vi "stepper driver -- progress monitor.vi"(8 "talkback user event":refnum<user-event>, 11 "talkto user event":refnum<user-event>) -> ()   [LabVIEW 2018]
uses:
  stepper motor state.ctl
  stepper progress monitor message.ctl
  talkto async routine action.ctl
  stepper driver action.ctl
  stepper driver -- BLM.vi
  stepper driver -- IMS.vi
panel:
  in  "stepper state":T1=enum."stopped"
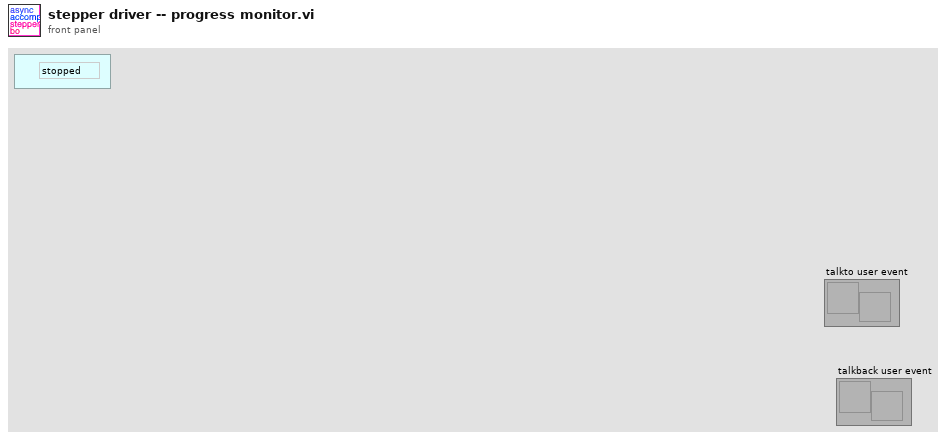
[diagram p1: front panel]
types:
  T1 = typedef "stepper motor state.ctl" = enum16{"moving", "stopped"}
  T2 = typedef "talkto async routine action.ctl" = enum16{"stop", "check"}
  T3 = typedef "stepper driver action.ctl" = enum16{"go", "void", "stop", "check", "init", "sync", "set", "set speed", "--check status", "--check value"}
  T4 = typedef "stepper progress monitor message.ctl" = cluster{"current position":dbl, "stepper motor state OUT":T1}
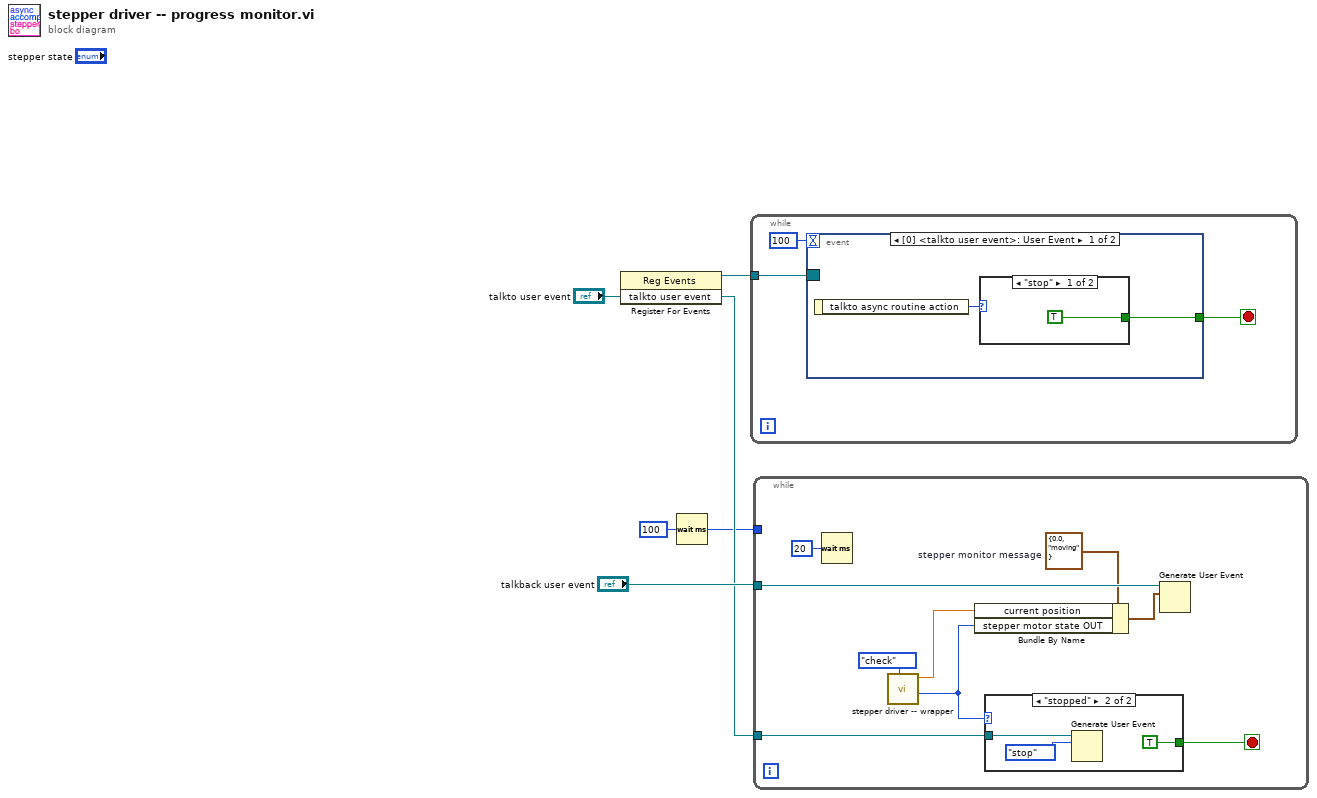
[diagram p0: block diagram]
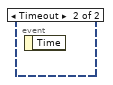
[diagram p3: hidden frame]
diagram:
  n1 = register-events("talkto user event") -> (reference out=w3:refnum<event-registration>)  [unwired: 2 in, 1 out]
  n2 = Wait (ms)(milliseconds to wait=u32 100) -> (millisecond timer value=w1:u32)
  n3 = while {
    tunnel: w3 -> [w8]
    stop <- w6 stop-if-true
    n4 = event shown="[0] <talkto user event>: User Event" {
      selector: w8 -> [_ _]
      dyn-events: _ -> [_ _]
      timeout: 100 -> [_ _]
      tunnel: [w9 _] -> w6
      event User Event {
        n5 = event-data() -> ("talkto async routine action"=w10:T2)  [unwired: 1 in]
        n6 = case shown="\"stop\"" w10 {
          tunnel: [TRUE _] -> w9
          frame "stop" {
          }
          frame "check", Default {
          }
        }
      }
      event Timeout {
        n7 = event-data() -> ()  [unwired: 1 in, 1 out]
      }
    }
  }
  n8 = while {
    tunnel: "talkback user event" -> [w20]
    tunnel: "talkto user event" -> [w19]
    tunnel: w1 -> [_]
    stop <- w18 stop-if-true
    w15 = T4 {"current position"=0.0, "stepper motor state OUT"=enum."moving"}  # stepper monitor message
    # "This loop is a consumer loop."
    n9 = Wait (ms)(milliseconds to wait=u32 20) -> ()  [unwired: 1 out]
    n10 = call "stepper driver -- wrapper.vi"("stepper driver action"=stepper_driver_action."check") -> ("stepper motor state OUT"=w12:T1, "number OUT"=w13:dbl)  [unwired: 8 in, 1 out]
    n11 = Bundle By Name(cluster=w15, "current position"=w13, "stepper motor state OUT"=w12) -> (w16:T4)
    n12 = case shown="\"stopped\"" w12 {
      tunnel: w19 -> [_ w23]
      tunnel: [_ TRUE] -> w18
      frame "moving", Default {
      }
      frame "stopped" {
        n13 = Generate User Event(user event=w23, event data cluster=talkto_async_routine_action."stop" ("event data")) -> ()  [unwired: 2 in, 2 out]
      }
    }
    n14 = Generate User Event(user event=w20, event data cluster=w16) -> ()  [unwired: 2 in, 2 out]
  }
